vi "Pose_TransformBy.vi"(9 "other TRANSFORM":T4, 11 "in POSE":T1) -> (3 "out POSE":T1)   [LabVIEW 2019, in "Trajectory_Library.lvlib"]
doc: "Transforms the pose by the given transformation and returns the new transformed pose. \"plus\" is the same as \"transformBy\"\n\nThe matrix multiplication is as follows\n [x_new] [cos, -sin, 0][transform.x]\n [y_new] += [sin, cos, 0][transform.y]\n [t_new] [0, 0, 1][transform.t]\n\nParameters:\n - IN POSE - The input POSE data structure\n - OTHER TRANSFORM - The transform to transform the pose by.\n\nReturn:\n - OUT POSE - The transformed pose."
uses:
  Trajectory_Library.lvlib
  POSE2D.ctl
  TRANSLATION2D.ctl
  ROTATION2D.ctl
  TRANSFORM2D.ctl
  Translation_Create.vi
  Rotation_RotateBy.vi
  Rotation_CreateXY.vi
  Util_CalcDist.vi
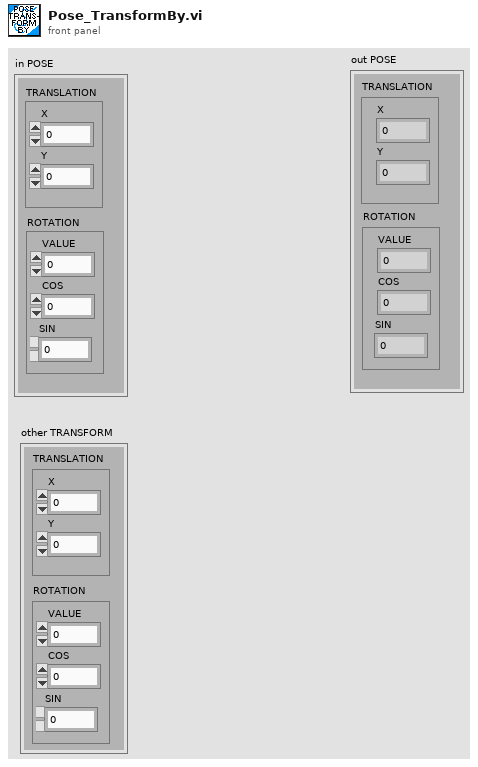
[diagram p1: front panel]
types:
  T1 = typedef "Trajectory_Library.lvlib/POSE2D.ctl" = cluster{"TRANSLATION":T2, "ROTATION":T3}
  T2 = typedef "Trajectory_Library.lvlib/TRANSLATION2D.ctl" = cluster{"X":dbl, "Y":dbl}
  T3 = typedef "Trajectory_Library.lvlib/ROTATION2D.ctl" = cluster{"VALUE":dbl, "COS":dbl, "SIN":dbl}
  T4 = typedef "Trajectory_Library.lvlib/TRANSFORM2D.ctl" = cluster{"TRANSLATION":T2, "ROTATION":T3}
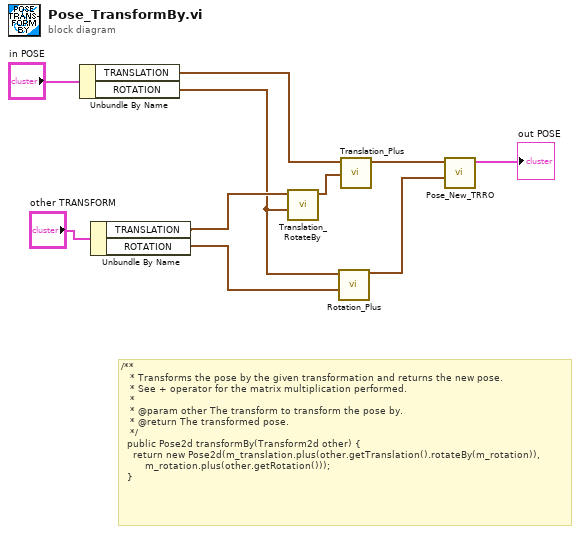
[diagram p0: block diagram]
diagram:
  # "/**\n   * Transforms the pose by the given transformation and returns the new pose.\n   * See + operator for the matrix multiplication performed.\n   *\n   * @param other The transform to transform the pose by.\n   * @return The transformed pose.\n   */\n  public Pose2d transformBy(Transform2d other) {\n    return new Pose2d(m_translation.plus(other.getTranslation().rotateBy(m_rotation)),\n        m_rotation.plus(other.getRotation()));\n  }"
  n1 = Unbundle By Name("in POSE") -> ("TRANSLATION"=w6:T2, "ROTATION"=w5:T3)
  n2 = Unbundle By Name("other TRANSFORM") -> ("TRANSLATION"=w8:T2, "ROTATION"=w4:T3)
  n3 = call "Translation_RotateBy.vi"("other Rotation"=w5, "In Translation"=w8) -> ("Out Translation"=w7:T2)  [unwired: 9 in]
  n4 = call "Rotation_Plus.vi"("other ROTATION"=w4, "in ROTATION"=w5) -> ("out ROTATION"=w2:T3)  [unwired: 9 in]
  n5 = call "Translation_Plus.vi"("other Translation"=w7, "In Translation"=w6) -> ("Out Translation"=w3:T2)  [unwired: 9 in]
  n6 = call "Pose_New_TRRO.vi"("ROTATION"=w2, "TRANSLATION"=w3) -> ("outPOSE"=→"out POSE":T1)  [unwired: 9 in]
